vi "ROS2 Write.vi"(9 "Data in":dbl[](array[numeric]), 10 "DDS":u64[](array[numeric]), 11 "error in":errorcluster[](array[cluster])) -> (2 "error out":errorcluster[](array[cluster]), 3 "DDS out":u64[](array[numeric]))   [LabVIEW 2021]
uses:
  <vilib>/RTI DDS Toolkit/VIs/Write_NumI32.vi
  <vilib>/RTI DDS Toolkit/Library/LVDDS_library.lvlib
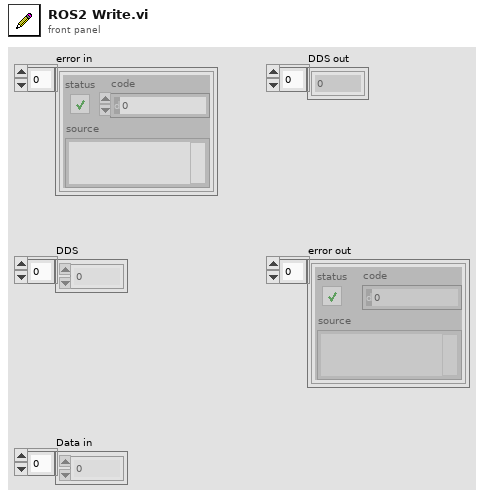
[diagram p1: front panel]
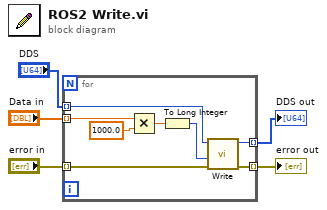
[diagram p0: block diagram]
diagram:
  n1 = for {
    tunnel: [w13] -> w2 mode=indexing
    tunnel: [w12] -> w4 mode=indexing
    tunnel: "DDS" -> [w8] mode=indexing
    tunnel: "error in" -> [w7] mode=indexing
    tunnel: "Data in" -> [w6] mode=indexing
    n2 = Multiply(x=w6, y=1000.0) -> (x*y=w11:dbl)
    n3 = To Long Integer(number=w11) -> (32bit integer=w9:i32)
    n4 = call-poly <vilib>:"Write.vi"("error in (no error)"=w7, "Data"=w9, "DDS Object Ref in"=w8) -> ("error out"=w12:errorcluster, "DDS Object Ref out"=w13:u64)  [unwired: 7 in]
  }
  "error out" <- w4
  "DDS out" <- w2
